vi "Indent.vi"(1 "Numeric":i32) -> (0 "string":string)   [LabVIEW 2009, in "Caraya.lvlib" / "Test Report.Default.lvclass"]
uses:
  Test Report.Default.lvclass
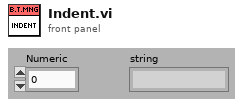
[diagram p1: front panel]
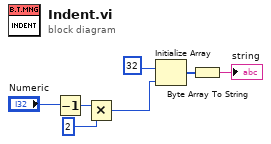
[diagram p0: block diagram]
diagram:
  n1 = Decrement(x="Numeric") -> (x-1=w2:i32)
  n2 = Multiply(x=w2, y=2) -> (x*y=w4:i32)
  n3 = Initialize Array(u8 32, w4) -> (w6:u8[])
  n4 = Byte Array To String(unsigned byte array=w6) -> (string=→"string":string)
